vi "go home.vi"(0 "ID in":i32) -> ()   [LabVIEW 2012]
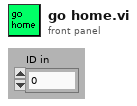
[diagram p1: front panel]
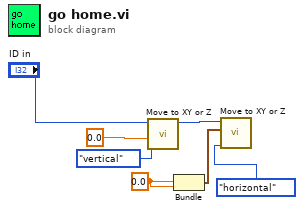
[diagram p0: block diagram]
diagram:
  w7 = dbl[unit] 0.0 ("y")
  n1 = call "Move to XY or Z.vi"("move type"=enum16{"horizontal", "vertical"}."vertical", "Z"=dbl[unit] 0.0, "ID"="ID in") -> ("ID out"=w1:i32)  [unwired: 7 in, 1 out]
  n2 = Bundle("y"=w7, "y"=w7) -> (w6:cluster{"y":dbl[unit], "y":dbl[unit]})  [unwired: 1 in]
  n3 = call "Move to XY or Z.vi"("move type"=enum16{"horizontal", "vertical"}."horizontal", "position 1"=w6, "ID"=w1) -> ()  [unwired: 7 in, 2 out]
